vi "auxilary.vi"() -> ()   [LabVIEW 2017]
uses:
  <vilib>/addons/Modulation/Analog/support/mod_Set Error Source.vi
  <vilib>/addons/Modulation/Digital/Support/Common/Validators/mod_Generate Filter Coefficients Validate.vi
  <vilib>/addons/Modulation/Digital/General/subVIs/mod_Generate Filter Coefficients.vi
  <vilib>/addons/Modulation/niDMT.lvlib
  <vilib>/Analysis/NI_AALPro.lvlib
panel:
  out "Array":u32[][](array[numeric])
  in  "String":string="1\t1\t2\t8\t9\t10\t15\t8\t10\t16\t2\t7\t15\t7\t16\n1\t1\t5\t16\t7\t3\t14\t16\t3\t10\t5\t12\t14\t12\t10\n1\t2\t1\t15\t5\t5\t12\t16\t6\t11\t2\t16\t11\t15\t12\n1\t2\t3\t1\t8\t6\t5\t2\t5\t8\t4\t4\t6\t3\t7\n1\t2\t16\t6\t6\t11\t15\t5\t12\t1\t15\t12\t16\t11\t2\n1\t3\t4\t7\t4\t1\t5\t5\t3\t6\t2\t8\t7\t6\t8\n1\t4\t11\t3\t4\t10\t9\t2\t11\t2\t10\t12\t12\t9\t3\n1\t5\t6\t6\t14\t9\t10\t2\t13\t9\t2\t5\t14\t1\t13\n1\t6\t10\t10\t4\t11\t7\t13\t16\t11\t13\t6\t4\t1\t16\n1\t6\t13\t2\t14\t2\t6\t5\t5\t13\t10\t9\t1\t14\t10\n1\t7\t8\t5\t7\t2\t4\t3\t8\t3\t2\t6\t6\t4\t5\n1\t7\t10\t9\t16\t7\t9\t15\t1\t8\t16\t8\t15\t2\t2\n1\t8\t12\t9\t9\t4\t13\t16\t5\t1\t13\t5\t12\t4\t8\n1\t8\t14\t10\t14\t1\t15\t15\t8\t5\t11\t4\t10\t5\t4\n1\t9\t2\t15\t15\t16\t10\t7\t8\t1\t10\t8\t2\t16\t9\n1\t9\t15\t6\t16\t2\t13\t14\t10\t11\t7\t4\t5\t12\t3\n1\t10\t9\t11\t15\t7\t6\t4\t16\t5\t2\t12\t13\t3\t14\n1\t11\t14\t4\t13\t2\t9\t10\t12\t16\t8\t5\t3\t15\t6\n1\t12\t12\t13\t14\t7\t2\t8\t14\t2\t1\t13\t11\t8\t11\n1\t12\t15\t5\t4\t14\t3\t16\t7\t8\t6\t2\t10\t11\t13\n1\t15\t4\t3\t7\t6\t10\t13\t12\t5\t14\t16\t8\t2\t11\n1\t16\t3\t12\t11\t9\t13\t5\t8\t2\t14\t7\t4\t10\t15\n2\t2\t5\t10\t16\t11\t3\t10\t11\t8\t5\t13\t3\t13\t8\n2\t2\t12\t3\t15\t5\t8\t3\t5\t14\t12\t9\t8\t9\t14\n2\t3\t6\t16\t12\t16\t3\t13\t13\t6\t7\t9\t2\t12\t7\n2\t3\t8\t2\t9\t15\t14\t3\t14\t9\t5\t5\t15\t8\t12\n2\t4\t7\t9\t5\t4\t9\t11\t2\t14\t5\t14\t11\t16\t16\n2\t4\t13\t12\t12\t7\t15\t10\t5\t2\t15\t5\t13\t7\t4\n2\t5\t9\t9\t3\t12\t8\t14\t15\t12\t14\t5\t3\t2\t15\n2\t5\t11\t7\t2\t11\t9\t4\t16\t7\t16\t9\t14\t14\t4\n2\t6\t2\t13\t3\t3\t12\t9\t7\t16\t6\t9\t16\t13\t12\n2\t6\t9\t7\t7\t16\t13\t3\t12\t2\t13\t12\t9\t16\t6\n2\t7\t12\t15\t2\t12\t4\t10\t13\t15\t13\t4\t5\t5\t10\n2\t7\t14\t16\t5\t9\t2\t9\t16\t11\t11\t5\t7\t4\t14\n2\t8\t5\t12\t5\t2\t14\t14\t8\t15\t3\t9\t12\t15\t9\n2\t9\t13\t4\t2\t13\t8\t11\t6\t4\t6\t8\t15\t15\t11\n2\t10\t3\t2\t13\t16\t8\t10\t8\t13\t11\t11\t16\t3\t5\n2\t11\t15\t3\t11\t6\t14\t10\t15\t10\t6\t7\t7\t14\t3\n2\t16\t4\t5\t16\t14\t7\t11\t4\t11\t14\t9\t9\t7\t5\n3\t3\t4\t6\t11\t12\t13\t6\t12\t14\t4\t5\t13\t5\t14\n3\t3\t6\t5\t16\t9\t15\t5\t9\t10\t6\t4\t15\t4\t10\n3\t4\t5\t14\t4\t6\t12\t13\t5\t13\t6\t11\t11\t12\t14\n3\t4\t9\t16\t10\t4\t16\t15\t3\t5\t10\t5\t15\t6\t6\n3\t4\t16\t10\t5\t10\t4\t9\t9\t16\t15\t6\t3\t5\t15\n3\t5\t12\t11\t14\t5\t11\t13\t3\t6\t14\t6\t13\t4\t4\n3\t6\t4\t10\t6\t5\t9\t15\t4\t15\t5\t16\t16\t9\t10\n3\t7\t8\t8\t16\t11\t12\t4\t15\t11\t4\t7\t16\t3\t15\n3\t7\t16\t11\t4\t15\t3\t15\t11\t12\t12\t4\t7\t8\t16\n3\t8\t7\t15\t4\t8\t15\t12\t3\t16\t4\t16\t12\t11\t11\n3\t8\t15\t4\t16\t4\t8\t7\t7\t15\t12\t11\t3\t16\t12\n3\t10\t10\t15\t16\t5\t4\t6\t16\t4\t3\t15\t9\t6\t9\n3\t13\t11\t5\t4\t12\t4\t11\t6\t6\t5\t3\t14\t13\t12\n3\t14\t7\t9\t14\t10\t13\t8\t7\t8\t10\t4\t4\t13\t9\n5\t5\t8\t14\t16\t13\t6\t14\t13\t7\t8\t15\t6\t15\t7\n5\t6\t11\t7\t10\t8\t5\t8\t7\t12\t12\t10\t6\t9\t11\n5\t6\t13\t8\t13\t5\t7\t7\t6\t16\t14\t15\t8\t16\t15\n5\t7\t9\t10\t7\t11\t6\t12\t9\t12\t11\t8\t8\t6\t10\n5\t9\t6\t8\t10\t9\t8\t12\t5\t11\t10\t11\t12\t7\t7\n5\t10\t10\t12\t8\t11\t9\t7\t8\t9\t5\t12\t6\t7\t6\n5\t10\t12\t6\t5\t12\t8\t9\t7\t6\t7\t8\t11\t11\t9\n5\t13\t15\t15\t14\t8\t6\t7\t16\t8\t7\t13\t14\t5\t16\n9\t10\t13\t10\t11\t15\t15\t9\t16\t12\t14\t13\t16\t14\t11\n9\t11\t12\t15\t12\t9\t13\t13\t11\t14\t10\t16\t15\t14\t16\n9\t12\t10\t15\t13\t14\t9\t14\t15\t11\t11\t13\t12\t16\t10\n"
  out "pulse shaping filter coefficients":dbl[](array[numeric]) format="%.2f"
  out "discr":cdb[](array[numeric])
  in  "I":cdb[](array[numeric])
  out "M2":i32[](array[numeric])
  out "M1":i32[](array[numeric])
  in  "width":i32=1000
  out "discriminator":dbl[](graph)
  out "Kd":dbl
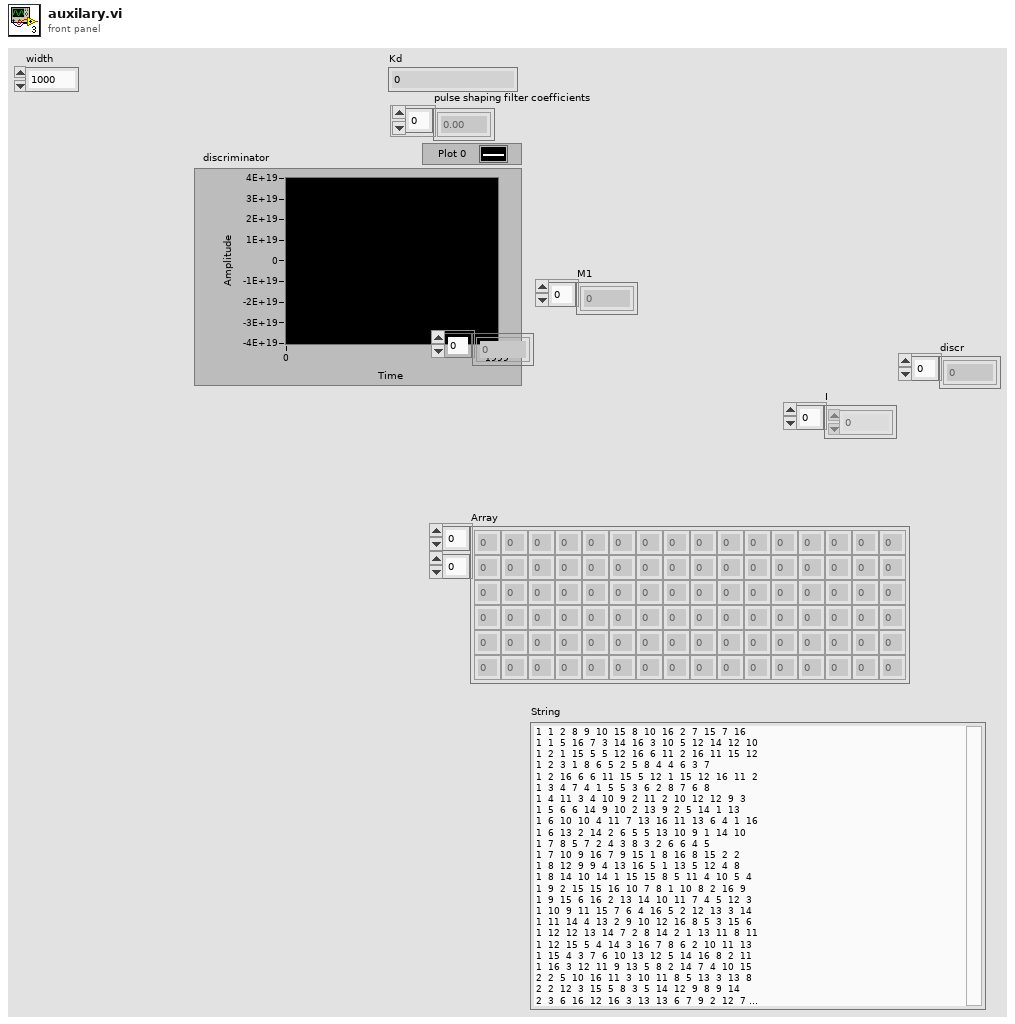
[diagram p1: front panel]
types:
  T1 = enum16{"none", "Raised Cosine", "Root Raised Cos", "Gaussian"}
  T2 = enum16{"FSK", "PSK", "QAM", "MSK", "PAM", "ASK", "CPM"}
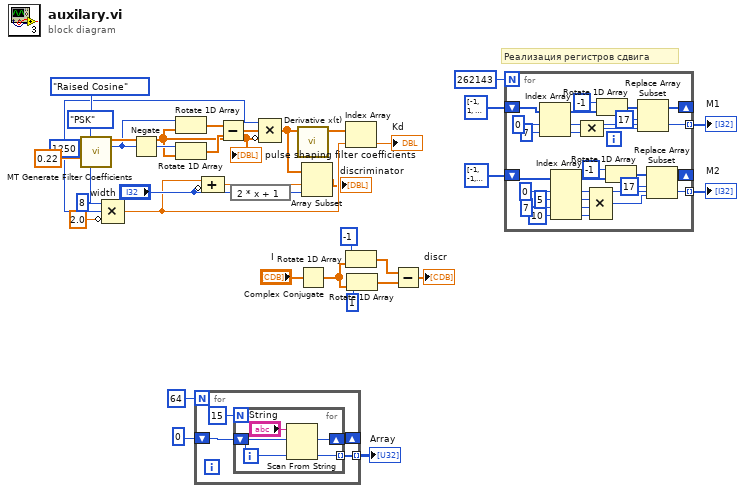
[diagram p0: block diagram]
diagram:
  w24 = 8 ("filter length (symbols)")
  w22 = 1250 ("pulse shaping samples per symbol (16)")
  # "Реализация регистров сдвига"
  n1 = call <vilib>:"MT Generate Filter Coefficients.vi"("pulse shaping filter (none)"=T1."Raised Cosine", "modulation type"=T2."PSK", "pulse shaping samples per symbol (16)"=w22, "filter parameter"=0.22, "filter length (symbols)"=w24) -> ("pulse shaping filter coefficients"=w25:dbl[])  [unwired: 8 in, 2 out]
  "pulse shaping filter coefficients" <- w25
  n2 = Compound Arithmetic op=MULTIPLY(w24, w22, invert 2.0 ("value")) -> (w17:dbl)
  n3 = Negate(x=w22) -> (-x=w29:i32)
  n4 = Rotate 1D Array(1:w25, 2:w22) -> (0:w31:dbl[])
  n5 = Rotate 1D Array(1:w25, 2:w29) -> (0:w30:dbl[])
  n6 = for {
    N: 64 -> [_]
    shift-right: [w37] -> _
    shift-left: 0 ("offset past number") -> [w36]
    tunnel: [w35] -> w2 mode=indexing
    n7 = for {
      N: 15 -> [_]
      shift-right: [w42] -> w37
      shift-left: w36 -> [w40]
      tunnel: [w41] -> w35 mode=indexing
      n8 = Scan From String(input string="String", initial scan location=w40, default 1=w40) -> (offset past scan=w42:u32, output 1=w41:u32)  [unwired: 2 in, 2 out]
    }
  }
  "Array" <- w2
  n9 = Compound Arithmetic op=unknown(w17, invert "width") -> (w20:dbl)
  n10 = Subtract(x=w31, y=w30) -> (x-y=w28:dbl[])
  n11 = expression code="2 * x + 1"("width") -> (w19:i32)
  n12 = Compound Arithmetic op=MULTIPLY(w22, w28, invert w25) -> (w21:dbl[])
  n13 = call <vilib>:"Derivative x(t).vi"("X"=w21) -> ("dX/dt"=w27:dbl[])  [unwired: 9 in, 1 out]
  n14 = Complex Conjugate(1:"I") -> (0:w4:cdb[])
  n15 = Array Subset(array=w21, index=w20, length=w19) -> (→"discriminator":dbl[])
  n16 = Index Array(array=w27, index=w17) -> (element=→"Kd":dbl)
  n17 = Rotate 1D Array(1:w4, 2:-1 ("n")) -> (0:w9:cdb[])
  n18 = Rotate 1D Array(1:w4, 2:1 ("n")) -> (0:w8:cdb[])
  n19 = Subtract(x=w9, y=w8) -> (x-y=→"discr":cdb[])
  n20 = for {
    N: 262143 -> [_]
    shift-right: [w63] -> _
    shift-left: i32[] [-1, 1, 1, 1, 1, 1, 1, 1, 1, 1, 1, 1, 1, 1, 1, 1, 1, 1] -> [w61]
    shift-right: [w50] -> _
    shift-left: i32[] [-1, -1, -1, -1, -1, -1, -1, -1, -1, -1, -1, -1, -1, -1, -1, -1, -1, -1] -> [w49]
    tunnel: [w44] -> w12 mode=indexing
    tunnel: [w43] -> w11 mode=indexing
    n21 = Index Array(array=w61, index #1=0 ("index"), index #2=7 ("index")) -> (element #1=w44:i32, element #2=w60:i32)
    n22 = Index Array(array=w49, index #1=0 ("index"), index #2=5 ("index"), index #3=7 ("index"), index #4=10 ("index")) -> (element #1=w43:i32, element #2=w53:i32, element #3=w48:i32, element #4=w47:i32)
    n23 = Compound Arithmetic op=MULTIPLY(w44, w60) -> (w62:i32)
    n24 = Compound Arithmetic op=MULTIPLY(w43, w53, w48, w47) -> (w54:i32)
    n25 = Rotate 1D Array(1:w61, 2:-1 ("n")) -> (0:w65:i32[])
    n26 = Rotate 1D Array(1:w49, 2:-1 ("n")) -> (0:w56:i32[])
    n27 = Replace Array Subset(array=w65, new element=w62, index=17) -> (w63:i32[])
    n28 = Replace Array Subset(array=w56, new element=w54, index=17) -> (w50:i32[])
  }
  "M1" <- w12
  "M2" <- w11
